vi "Set Run State.vi"(8 "error in (no error)":errorcluster, 10 "RunState(T)":bool=TRUE, 11 "reference in":refnum<k24>) -> (0 "error out":errorcluster, 3 "reference out":refnum<k24>)   [LabVIEW 2019, in "LabNation Scope Driver.lvlib"]
doc: "Sets the run state of the Scope."
uses:
  LabNation Scope Driver.lvlib
  C:/Program Files (x86)/LabNation/SmartScope/DeviceInterface.dll
  Program Files (x86)/LabNation/SmartScope/DeviceInterface.dll
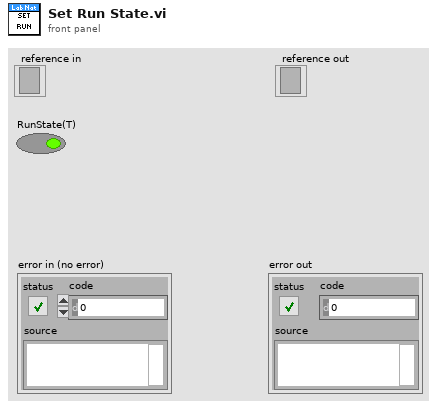
[diagram p1: front panel]
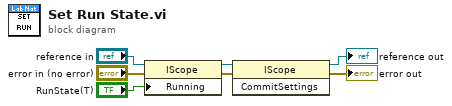
[diagram p0: block diagram]
diagram:
  n1 = property class="IScope"(reference="reference in", error in="error in (no error)", "Running"="RunState(T)") -> (reference out=w7:refnum<k24>, error out=w5:errorcluster)
  n2 = invoke class="IScope" method="CommitSettings"(reference=w7, error in=w5) -> (reference out=→"reference out":refnum<k24>, error out=→"error out":errorcluster)  [unwired: 1 in, 1 out]
